vi "test chunkloader.vi"() -> ()   [LabVIEW 2014]
panel:
  in  "Size":i32[](array[numeric])
  out "appended array":dbl[][][][](array[numeric])
  in  "Array":dbl[][][][](array[numeric])
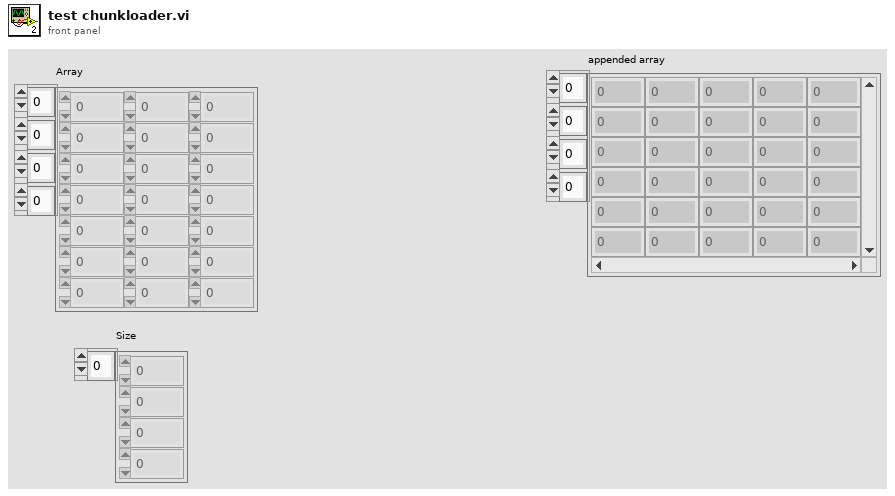
[diagram p1: front panel]
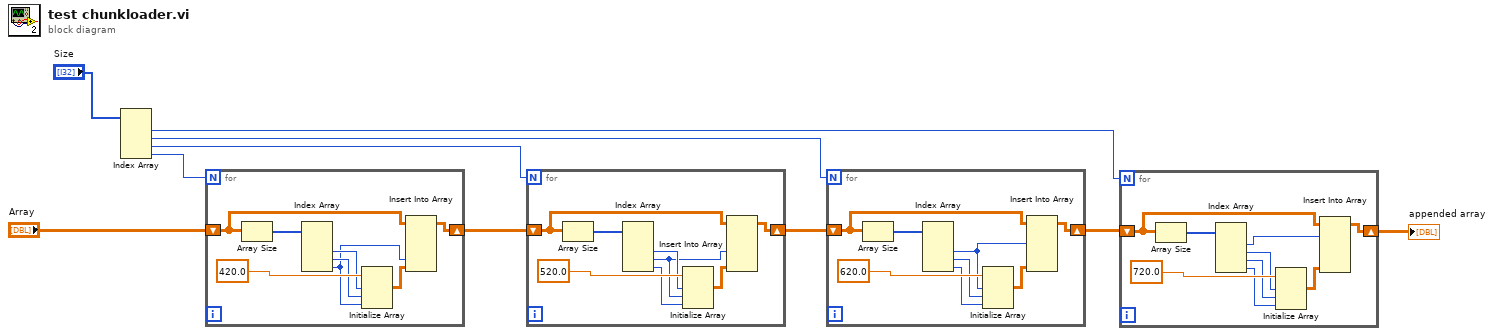
[diagram p0: block diagram]
diagram:
  n1 = Index Array(array="Size") -> (element #1=w2:i32, element #2=w4:i32, element #3=w6:i32, element #4=w7:i32)  [unwired: 4 in]
  n2 = for {
    N: w7 -> [_]
    shift-right: [w18] -> w8
    shift-left: "Array" -> [w15]
    n3 = Array Size(array=w15) -> (size(s)=w17:i32[])
    n4 = Index Array(array=w17) -> (element #2=w12:i32, element #3=w13:i32, element #4=w11:i32)  [unwired: 4 in, 1 out]
    n5 = Initialize Array(420.0 ("element"), w12, w13, w11) -> (w16:dbl[][][])
    n6 = Insert Into Array(array=w15, index (dim 3)=w11, new element=w16) -> (w18:dbl[][][][])  [unwired: 3 in]
  }
  n7 = for {
    N: w6 -> [_]
    shift-right: [w26] -> w5
    shift-left: w8 -> [w23]
    n8 = Array Size(array=w23) -> (size(s)=w25:i32[])
    n9 = Index Array(array=w25) -> (element #2=w20:i32, element #3=w19:i32, element #4=w21:i32)  [unwired: 4 in, 1 out]
    n10 = Initialize Array(520.0 ("element"), w20, w19, w21) -> (w24:dbl[][][])
    n11 = Insert Into Array(array=w23, index (dim 2)=w19, new element=w24) -> (w26:dbl[][][][])  [unwired: 3 in]
  }
  n12 = for {
    N: w4 -> [_]
    shift-right: [w34] -> w3
    shift-left: w5 -> [w31]
    n13 = Array Size(array=w31) -> (size(s)=w33:i32[])
    n14 = Index Array(array=w33) -> (element #2=w27:i32, element #3=w29:i32, element #4=w28:i32)  [unwired: 4 in, 1 out]
    n15 = Initialize Array(620.0 ("element"), w27, w29, w28) -> (w32:dbl[][][])
    n16 = Insert Into Array(array=w31, index (dim 1)=w27, new element=w32) -> (w34:dbl[][][][])  [unwired: 3 in]
  }
  n17 = for {
    N: w2 -> [_]
    shift-right: [w43] -> w1
    shift-left: w3 -> [w40]
    n18 = Array Size(array=w40) -> (size(s)=w42:i32[])
    n19 = Index Array(array=w42) -> (element #1=w35:i32, element #2=w38:i32, element #3=w37:i32, element #4=w36:i32)  [unwired: 4 in]
    n20 = Initialize Array(720.0 ("element"), w38, w37, w36) -> (w41:dbl[][][])
    n21 = Insert Into Array(array=w40, index (dim 0)=w35, new element=w41) -> (w43:dbl[][][][])  [unwired: 3 in]
  }
  "appended array" <- w1
